vi "FTW-ActorTemplate.vi"(0 "Actor Instance Configuration":string="{\n  \"Identity\": \"ActorName\",\n  \"InboxAddress\": \"tcp://127.0.0.1:*\",\n  \"SupervisorAddress\": \"\",\n  \"DebugEnableInboxLogging\": false,\n  \"DebugEnableJobLogging\": false,\n  \"DebugShowPanel\": false\n}", 11 "ErrorIn":errorcluster) -> (15 "Error":errorcluster)   [LabVIEW 2015]
uses:
  src/actor/instance/FTW-Actor-Instance.lvclass
panel:
  # "Inputs"
  # "Outputs"
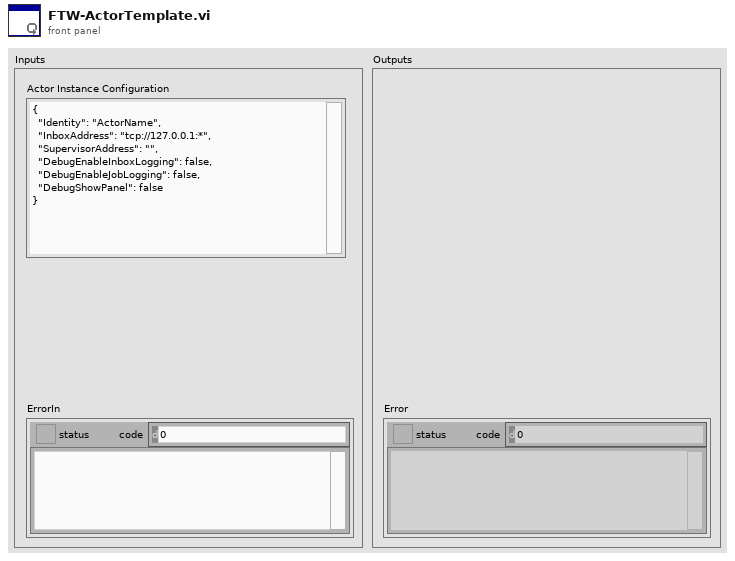
[diagram p1: front panel]
types:
  T1 = cluster{"Incoming Request":refnum<event-registration>}
  T2 = typedef "FTW-Type-JSON.ctl" = refnum<data-value>
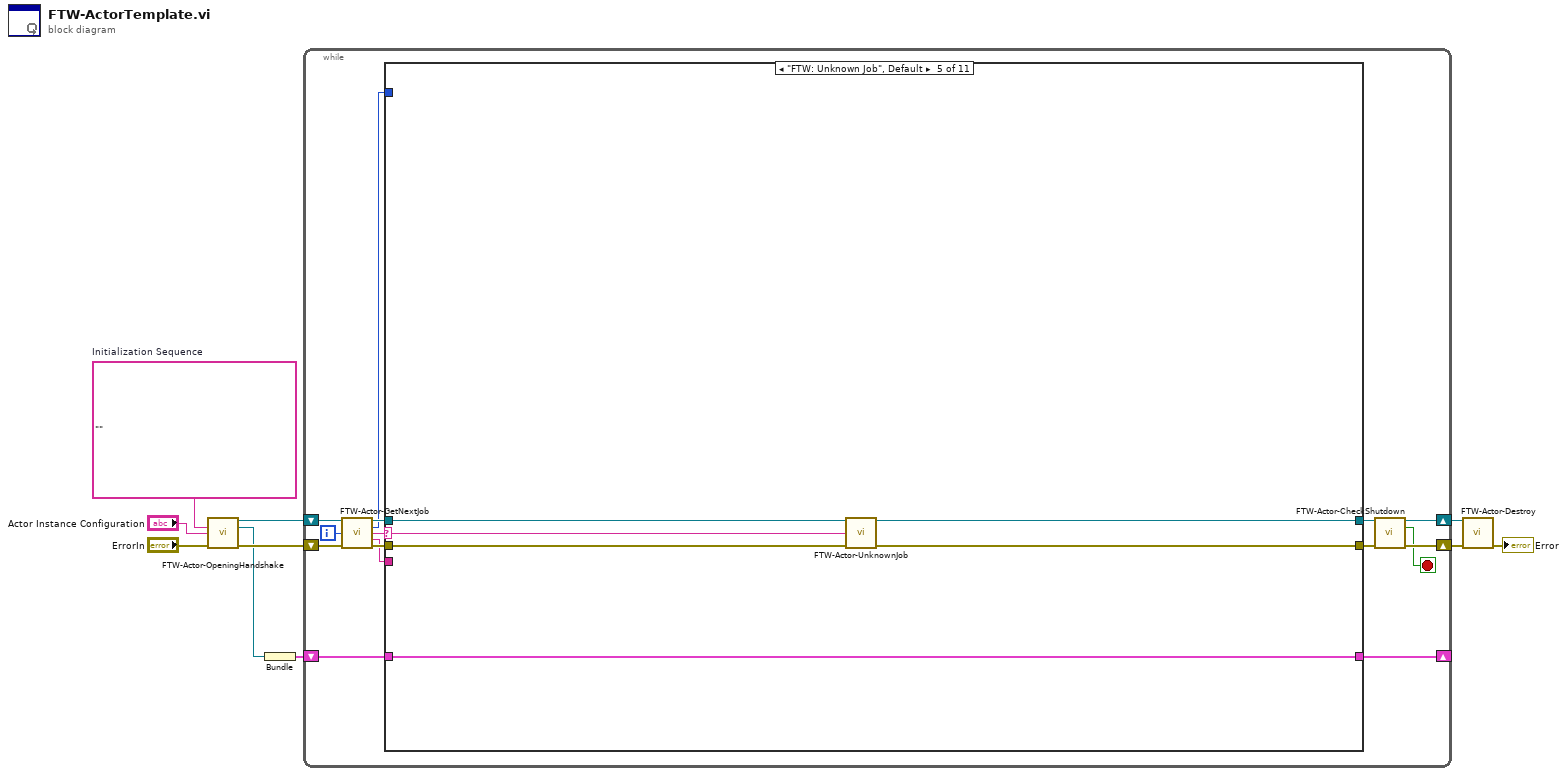
[diagram p0: block diagram]
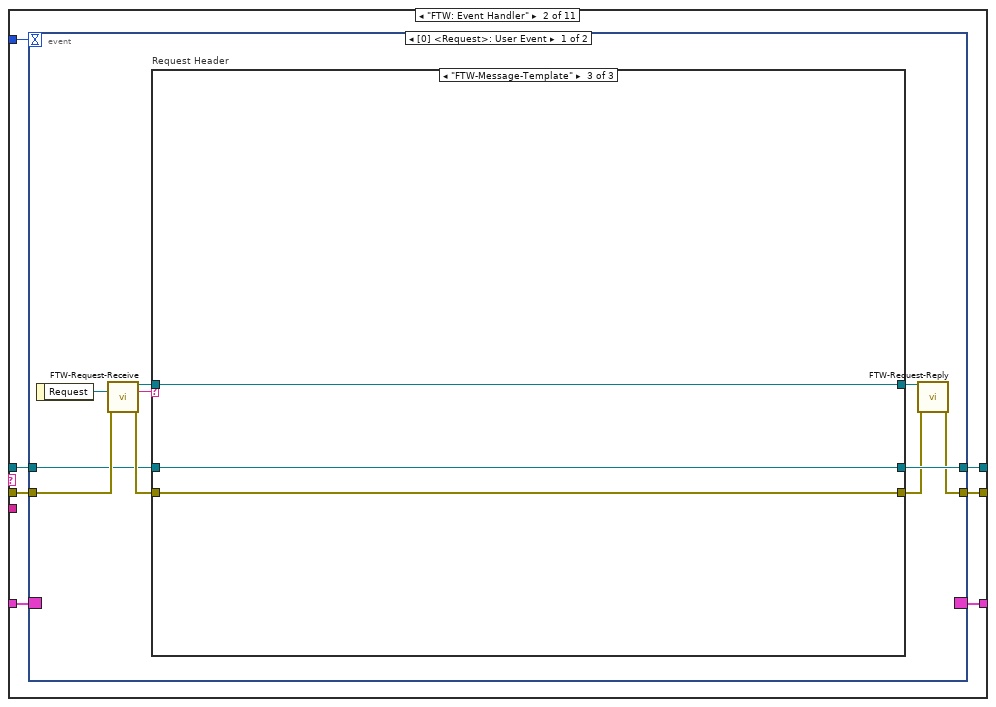
[diagram p3: hidden frame]
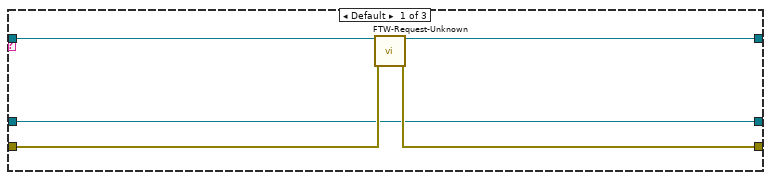
[diagram p4: hidden frame]
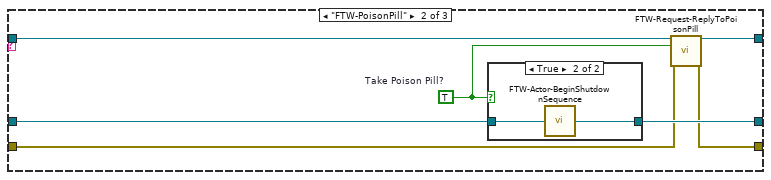
[diagram p5: hidden frame]
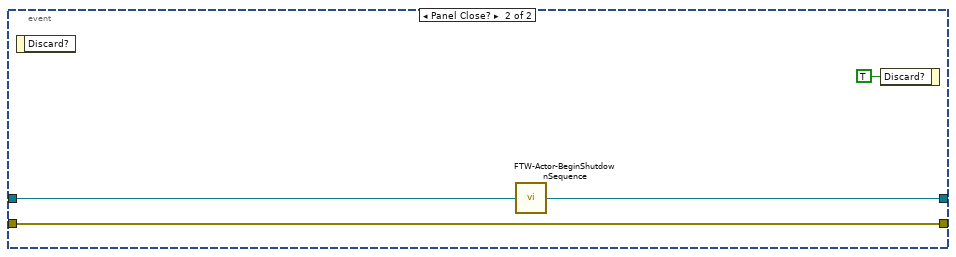
[diagram p7: hidden frame]
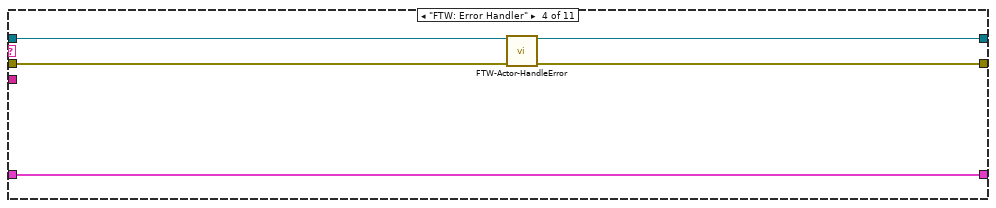
[diagram p9: hidden frame]
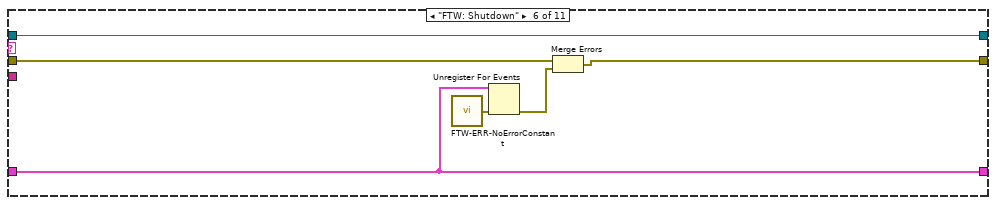
[diagram p10: hidden frame]
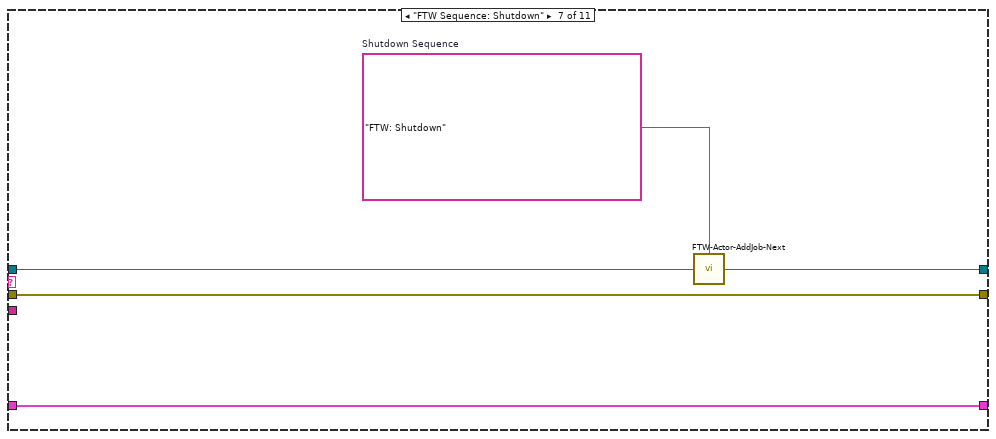
[diagram p11: hidden frame]
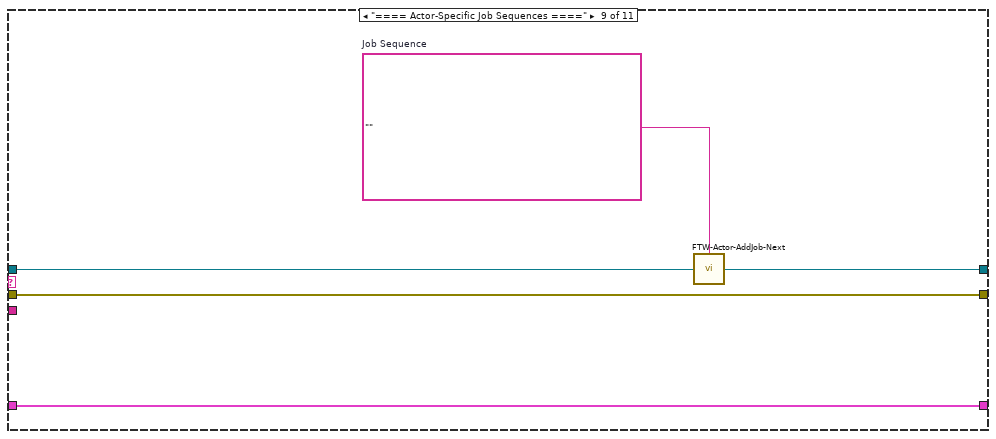
[diagram p13: hidden frame]
diagram:
  w5 = ""  # Initialization Sequence
  n1 = call "FTW-Actor-OpeningHandshake.vi"("Initialization Job Sequence"=w5, "Actor Instance Configuration"="Actor Instance Configuration", "error in"="ErrorIn") -> ("FTW Actor Instance"=w10:refnum<class "FTW-Actor-Instance.lvclass">, "Incoming Request"=w1:refnum<event-registration>, "error out"=w6:errorcluster)  [unwired: 10 in]
  n2 = Bundle("Incoming Request"=w1) -> (w3:T1)  [unwired: 1 in]
  n3 = while {
    shift-right: [w15] -> w8
    shift-left: w6 -> [w22]
    shift-right: [w12] -> _
    shift-left: w3 -> [w25]
    shift-right: [w17] -> w9
    shift-left: w10 -> [w24]
    i -> [w13]
    stop <- w14 stop-if-true
    n4 = call "FTW-Actor-GetNextJob.vi"("FTW Actor Instance"=w24, "Jobs Performed"=w13, "error in"=w22) -> ("FTW Actor Instance out"=w23:refnum<class "FTW-Actor-Instance.lvclass">, "Event Structure Timeout"=w11:i32, "Job Name"=w20:string, "Job Data"=w19:string, "error out"=w21:errorcluster)  [unwired: 8 in]
    n5 = case shown="\"FTW: Unknown Job\", Default" w20 {
      selector: w20 -> [_ _ _ _ w76 _ _ _ _ _ _]
      tunnel: [w27 w35 w68 w71 w79 w86 w91 w94 w99 w103 w106] -> w16
      tunnel: w21 -> [w27 w34 w68 w73 w80 w87 w91 w94 w99 w103 w106]
      tunnel: w25 -> [w28 w30 w70 w75 w81 w83 w92 w95 w100 w102 w105]
      tunnel: [w28 w33 w70 w75 w81 w83 w92 w95 w100 w102 w105] -> w12
      tunnel: w19 -> [_ _ _ _ _ _ _ _ _ _ _]
      tunnel: [w26 w32 w69 w72 w77 w84 w89 w93 w97 w101 w104] -> w18
      tunnel: w23 -> [w26 w31 w69 w74 w78 w84 w90 w93 w98 w101 w104]
      tunnel: w11 -> [_ w29 _ _ _ _ _ _ _ _ _]
      frame "==== Featherweight Framework Jobs ====" {
      }
      frame "FTW: Event Handler" {
        n6 = event shown="[0] <Request>: User Event" {
          selector: w30 -> [_ _]
          dyn-events: [_ _] -> w33
          timeout: w29 -> [_ _]
          tunnel: [w39 w66] -> w35
          tunnel: w34 -> [w44 w66]
          tunnel: [w43 w64] -> w32
          tunnel: w31 -> [w42 w65]
          event User Event {
            n7 = event-data() -> ("Request"=w36:refnum<queue>)  [unwired: 1 in]
            n8 = call "FTW-Request-Receive.vi"("MessagePipe"=w36, "error in"=w44) -> ("Request"=w40:T2, "Request Header"=w41:string, "error out"=w45:errorcluster)  [unwired: 11 in]
            n9 = case "Request Header" shown="\"FTW-Message-Template\"" w41 {
              tunnel: [w49 w52 w61] -> w38
              tunnel: w45 -> [w50 w53 w61]
              tunnel: [w47 w57 w63] -> w43
              tunnel: w42 -> [w47 w56 w63]
              tunnel: w40 -> [w48 w55 w62]
              tunnel: [w46 w54 w62] -> w37
              frame Default {
                n10 = call "FTW-Request-Unknown.vi"("Request"=w48, "error in"=w50) -> ("Request out"=w46:T2, "error out"=w49:errorcluster)  [unwired: 12 in]
              }
              frame "FTW-PoisonPill" {
                w51 = TRUE  # Take Poison Pill?
                n11 = case shown="True" w51 {
                  tunnel: [w58 w60] -> w57
                  tunnel: w56 -> [w58 w59]
                  frame False {
                  }
                  frame True {
                    n12 = call "FTW-Actor-BeginShutdownSequence.vi"("FTW Actor Instance"=w59) -> ("FTW Actor Instance out"=w60:refnum<class "FTW-Actor-Instance.lvclass">)  [unwired: 3 in]
                  }
                }
                n13 = call "FTW-Request-ReplyToPoisonPill.vi"("Poison Pill Request"=w55, "Shutting Down?"=w51, "error in"=w53) -> ("Poison Pill Response"=w54:T2, "error out"=w52:errorcluster)  [unwired: 11 in]
              }
              frame "FTW-Message-Template" {
              }
            }
            n14 = call "FTW-Request-Reply.vi"("Request"=w37, "error in"=w38) -> ("error out"=w39:errorcluster)  [unwired: 13 in]
          }
          event Panel Close? {
            n15 = event-data() -> ()  [unwired: 1 in, 1 out]
            n16 = call "FTW-Actor-BeginShutdownSequence.vi"("FTW Actor Instance"=w65) -> ("FTW Actor Instance out"=w64:refnum<class "FTW-Actor-Instance.lvclass">)  [unwired: 3 in]
            n17 = event-data("Discard?"=TRUE) -> ()  [unwired: 1 in, 1 out]
          }
        }
      }
      frame "FTW: Failure to Launch" {
      }
      frame "FTW: Error Handler" {
        n18 = call "FTW-Actor-HandleError.vi"("FTW Actor Instance"=w74, "error in"=w73) -> ("FTW Actor Instance out"=w72:refnum<class "FTW-Actor-Instance.lvclass">, "error out"=w71:errorcluster)  [unwired: 11 in, 1 out]
      }
      frame "FTW: Unknown Job", Default {
        n19 = call "FTW-Actor-UnknownJob.vi"("FTW Actor Instance"=w78, "Unknown Job"=w76, "error in"=w80) -> ("FTW Actor Instance out"=w77:refnum<class "FTW-Actor-Instance.lvclass">, "error out"=w79:errorcluster)  [unwired: 11 in]
      }
      frame "FTW: Shutdown" {
        n20 = call "FTW-ERR-NoErrorConstant.vi"() -> ("no error"=w82:errorcluster)
        n21 = Unregister For Events(event registration refnum=w83, error in=w82) -> (error out=w85:errorcluster)
        n22 = Merge Errors(w87, w85) -> (w86:errorcluster)
      }
      frame "FTW Sequence: Shutdown" {
        w88 = "FTW: Shutdown"  # Shutdown Sequence
        n23 = call "FTW-Actor-AddJob-Next.vi"("Add Next in Job Queue"=w88, "FTW Actor Instance"=w90) -> ("FTW Actor Instance out"=w89:refnum<class "FTW-Actor-Instance.lvclass">)  [unwired: 2 in]
      }
      frame "==== Actor-Specific Static Dependencies ====" {
      }
      frame "==== Actor-Specific Job Sequences ====" {
        w96 = ""  # Job Sequence
        n24 = call "FTW-Actor-AddJob-Next.vi"("Add Next in Job Queue"=w96, "FTW Actor Instance"=w98) -> ("FTW Actor Instance out"=w97:refnum<class "FTW-Actor-Instance.lvclass">)  [unwired: 2 in]
      }
      frame "==== Actor-Specific Jobs ====" {
      }
      frame "ActorName: Job Template" {
      }
    }
    n25 = call "FTW-Actor-CheckShutdown.vi"("FTW Actor Instance"=w18, "error in"=w16) -> ("FTW Actor Instance out"=w17:refnum<class "FTW-Actor-Instance.lvclass">, "Shutdown?"=w14:bool, "error out"=w15:errorcluster)  [unwired: 11 in]
  }
  n26 = call "FTW-Actor-Destroy.vi"("FTW Actor Instance"=w9, "error in"=w8) -> ("error out"=→"Error":errorcluster)  [unwired: 12 in, 1 out]
